vi "FXP_bitfile.vi"() -> ()   [LabVIEW 2018]
panel:
  out "RPM":fxp<+/-,16,5>
  in  "VALUE":fxp<+/-,16,5>=15.5
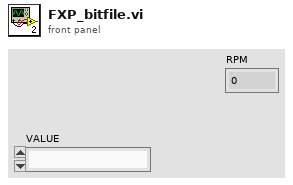
[diagram p1: front panel]
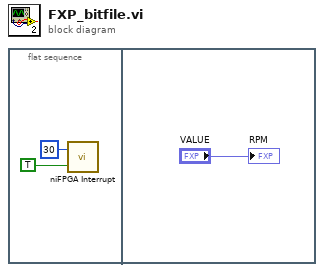
[diagram p0: block diagram]
diagram:
  n1 = flat-sequence {
    frame #0 {
      n2 = call <vilib>:"niFPGA Interrupt.vi"("Wait Until Cleared (F)"=TRUE, "IRQ Number (0)"=u8 30) -> ()  [unwired: 1 in]
    }
    frame #1 {
      "RPM" <- "VALUE"
    }
  }
